vi "set output trigger.vi"(8 "error in (no error)":errorcluster, 11 "DAQOrcaFlash in":refnum<class "DAQOrcaFlash.lvclass">) -> (0 "error out":errorcluster, 3 "DAQOrcaFlash out":refnum<class "DAQOrcaFlash.lvclass">)   [LabVIEW 2012, in "DAQOrcaFlash.lvclass"]
uses:
  DAQOrcaFlash.lvclass
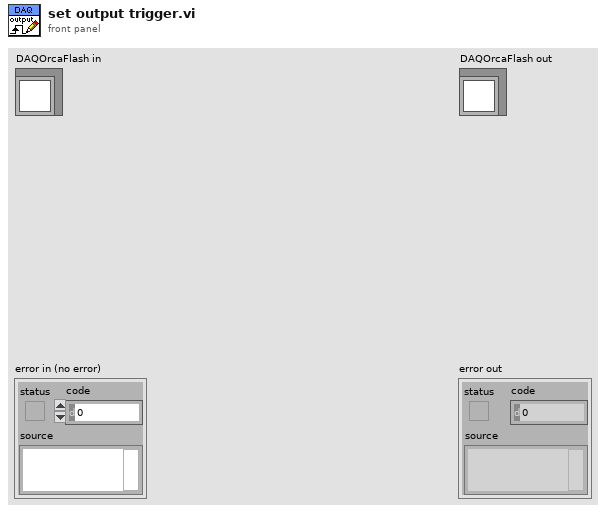
[diagram p1: front panel]
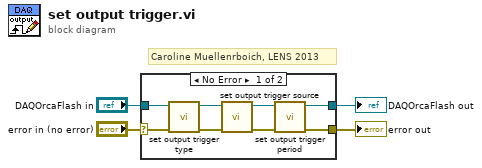
[diagram p0: block diagram]
diagram:
  # "Caroline Muellenrboich, LENS 2013"
  n1 = case shown="No Error" "error in (no error)" {
    selector: "error in (no error)" -> [w8 w14]
    tunnel: [w5 w14] -> w4
    tunnel: [w9 w13] -> w2
    tunnel: "DAQOrcaFlash in" -> [w12 w13]
    frame No Error {
      n2 = call-dynamic "set output trigger type.vi"("error in (no error)"=w8, "DAQOrcaFlash in"=w12) -> ("error out"=w7:errorcluster, "DAQOrcaFlash out"=w11:refnum<class "DAQOrcaFlash.lvclass">)  [unwired: 8 in]
      n3 = call-dynamic "set output trigger source.vi"("error in (no error)"=w7, "DAQOrcaFlash in"=w11) -> ("error out"=w6:errorcluster, "DAQOrcaFlash out"=w10:refnum<class "DAQOrcaFlash.lvclass">)  [unwired: 8 in]
      n4 = call-dynamic "set output trigger period.vi"("error in (no error)"=w6, "DAQOrcaFlash in"=w10) -> ("error out"=w5:errorcluster, "DAQOrcaFlash out"=w9:refnum<class "DAQOrcaFlash.lvclass">)  [unwired: 8 in]
    }
    frame Error {
    }
  }
  "error out" <- w4
  "DAQOrcaFlash out" <- w2
